vi "PV ASM340 Trigger.vi"(8 "error in (no error)":errorcluster, 9 "HLT 5xx Trigger - Cluster":T1={"Parameter"=0, "Parameter\nread only<->describe"=FALSE, "Trigger Twin Flow low"=5.0, "Trigger Twin Flow high"=0.5, "Trigger Counter Flow"=15.0} {"Trigger Counter Flow" min=0.1 max=25.0 step=0.1 format="%.2f"; "Trigger Twin Flow high" min=0.01 max=0.5 step=0.01 format="%.2f"; "Trigger Twin Flow low" min=0.1 max=5.0 step=0.1 format="%.2f"; "Parameter" items=[" Trigger Counter Flow", " Trigg Twin-Flow low", " Trigg Twin-Flow high"]}, 10 "Adress of unit":u16=1 min=1 max=999 step=1, 11 "VISA session":refnum<visa-resource-name>) -> (0 "error out":errorcluster, 2 "response (data)":string, 3 "dup VISA session":refnum<visa-resource-name>)   [LabVIEW 2021, in "Pfeiffer Vacuum.lvlib"]
doc: "There are 3 parameters available, only one of which can be enabled at a time. \n\n0 - Trigger Counter Flow - (default) Para 660\n1 - Trigger Twin Flow low - Para 661\n2 - Trigger Twin Flow high - Para 662\n\nNote: The 3 controls right of this one will set the appropriate values for the selected parameter. Any settings for an parameter that is not selected will be ignored. If a value is out of range, it will be changed to either the upper or the lower limit of the range."
uses:
  <instrlib>/Pfeiffer Vacuum/Pfeiffer Vacuum.lvlib
  <instrlib>/Pfeiffer Vacuum/Public/LeakDetector/LeakDetector Configure/PV HLT5xx Trigger.ctl
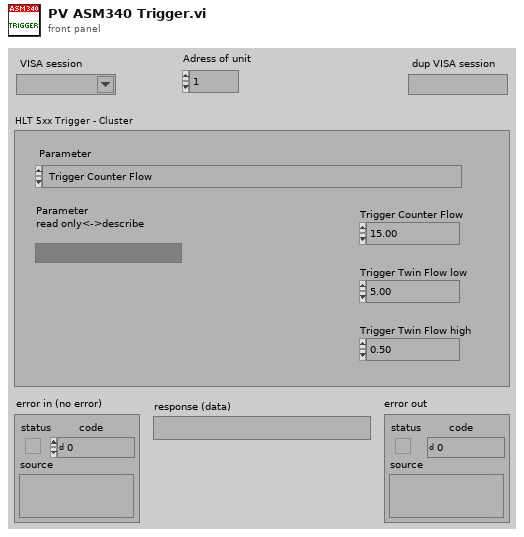
[diagram p1: front panel]
types:
  T1 = typedef "Pfeiffer Vacuum.lvlib/PV HLT5xx Trigger.ctl" = cluster{"Parameter":u16, "Parameter\nread only<->describe":bool, "Trigger Twin Flow low":dbl, "Trigger Twin Flow high":dbl, "Trigger Counter Flow":dbl}
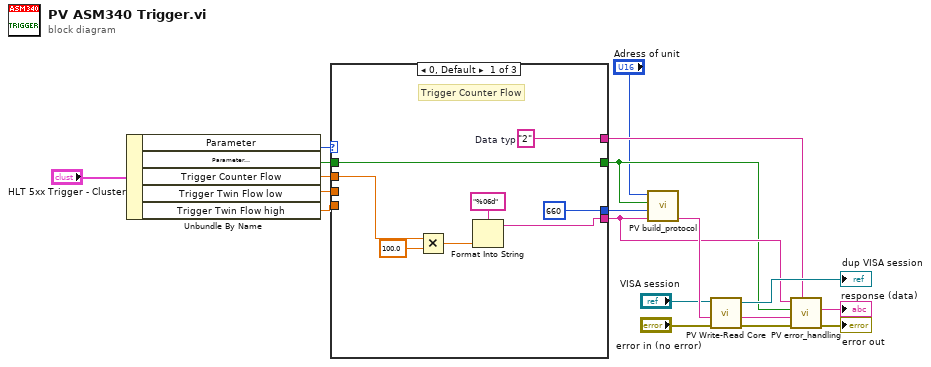
[diagram p0: block diagram]
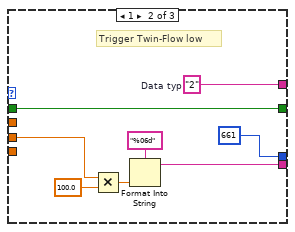
[diagram p2: hidden frame]
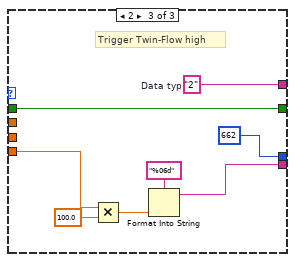
[diagram p3: hidden frame]
diagram:
  n1 = Unbundle By Name("HLT 5xx Trigger - Cluster") -> ("Parameter"=w6:u16, "Parameter\nread only<->describe"=w18:bool, "Trigger Counter Flow"=w4:dbl, "Trigger Twin Flow low"=w3:dbl, "Trigger Twin Flow high"=w2:dbl)
  n2 = case shown="0, Default" w6 {
    tunnel: [u16 660 ("Parameter-number") u16 661 ("Parameter-number") u16 662 ("Parameter-number")] -> w19
    tunnel: [w23 w31 w39] -> w13
    tunnel: [w24 w34 w42] -> w11
    tunnel: w18 -> [w24 w34 w42]
    tunnel: [w27 w35 w43] -> w12
    tunnel: w4 -> [w21 _ _]
    tunnel: w3 -> [_ w28 _]
    tunnel: w2 -> [_ _ w36]
    frame 0, Default {
      w27 = "2"  # Data typ
      # "Trigger Counter Flow"
      n3 = Multiply(x=w21, y=100.0) -> (x*y=w20:dbl)
      n4 = Format Into String(format string="%06d" ("Format-String"), w20) -> (resulting string=w23:string)  [unwired: 2 in, 1 out]
    }
    frame 1 {
      w35 = "2"  # Data typ
      # "Trigger Twin-Flow low"
      n5 = Multiply(x=w28, y=100.0) -> (x*y=w29:dbl)
      n6 = Format Into String(format string="%06d" ("Format-String"), w29) -> (resulting string=w31:string)  [unwired: 2 in, 1 out]
    }
    frame 2 {
      w43 = "2"  # Data typ
      # "Trigger Twin-Flow high"
      n7 = Multiply(x=w36, y=100.0) -> (x*y=w37:dbl)
      n8 = Format Into String(format string="%06d" ("Format-String"), w37) -> (resulting string=w39:string)  [unwired: 2 in, 1 out]
    }
  }
  n9 = call <instrlib>:"PV build_protocol.vi"("Data"=w13, "Parameter-number"=w19, "parameter\nread<->describe"=w11, "Adress"="Adress of unit") -> ("output"=w17:string)  [unwired: 3 in]
  n10 = call <instrlib>:"PV Write-Read Core.vi"("error in"="error in (no error)", "Write data in"=w17, "VISA session"="VISA session") -> ("error out"=w15:errorcluster, "response (data) out"=w16:string, "dup VISA session"=→"dup VISA session":refnum<visa-resource-name>)  [unwired: 2 in]
  n11 = call <instrlib>:"PV error_handling.vi"("Data Typ in"=w12, "error in"=w15, "response (data) in"=w16, "Parameter\nread only<->describe"=w11, "data in"=w13) -> ("error out"=→"error out":errorcluster, "Data out"=→"response (data)":string)  [unwired: 4 in, 1 out]
